vi "Upsampling for Reso Correction.vi"(9 "Insert Positions IN (for recursion)":i32[](array[numeric]), 10 "Extra points":i32, 11 "Pixel Map IN":i32[](array[numeric])) -> (2 "Insert Positions OUT":i32[](array[numeric]), 3 "Pixel Map OUT (Zoomed in)":i32[](array[numeric]))   [LabVIEW 2012]
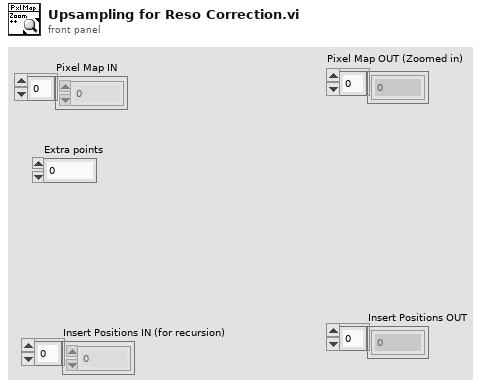
[diagram p1: front panel]
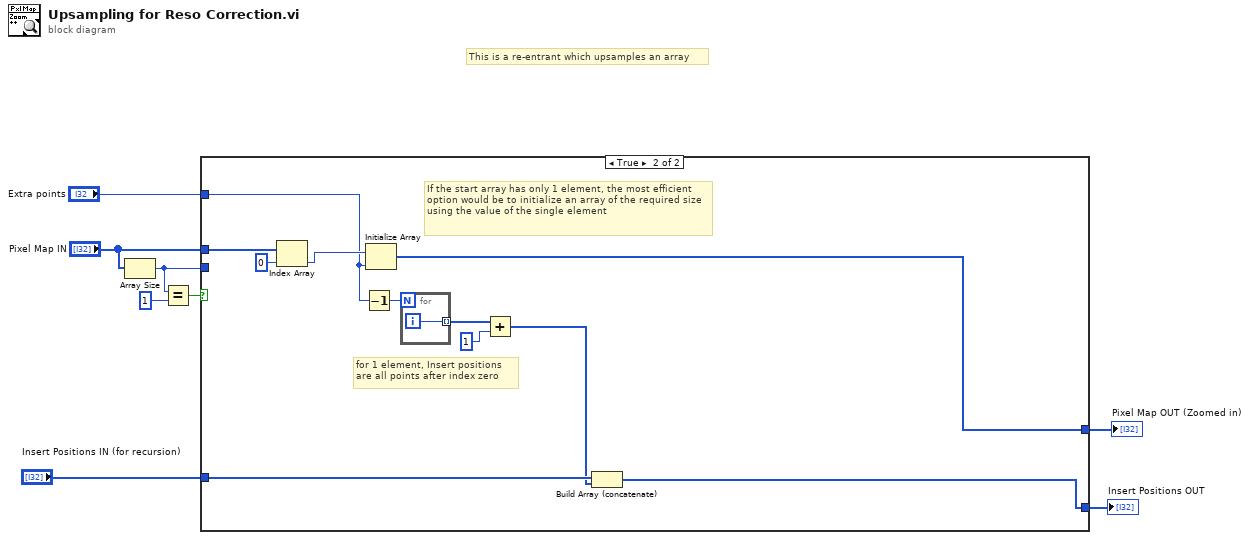
[diagram p0: block diagram]
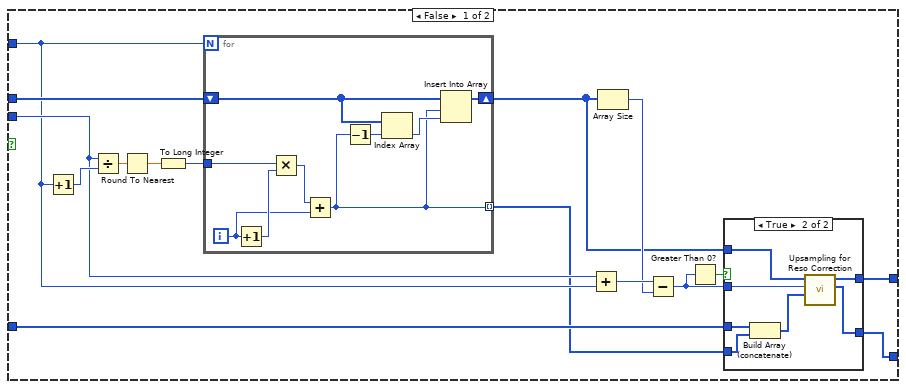
[diagram p2: hidden frame]
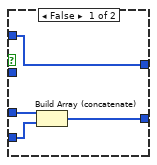
[diagram p3: hidden frame]
diagram:
  # "This is a re-entrant which upsamples an array"
  n1 = Array Size(array="Pixel Map IN") -> (size(s)=w5:i32)
  n2 = Equal?(x=w5, y=1) -> (x = y?=w3:bool)
  n3 = case shown="True" w3 {
    tunnel: w5 -> [w20 _]
    tunnel: "Pixel Map IN" -> [w14 w55]
    tunnel: "Extra points" -> [w13 w51]
    tunnel: [w12 w52] -> w6
    tunnel: [w9 w45] -> w2
    tunnel: "Insert Positions IN (for recursion)" -> [w11 w47]
    frame False {
      n4 = Increment(x=w13) -> (x+1=w24:i32)
      n5 = Divide(x=w20, y=w24) -> (x/y=w23:dbl)
      n6 = Round To Nearest(number=w23) -> (nearest integer value=w22:dbl)
      n7 = To Long Integer(number=w22) -> (32bit integer=w21:i32)
      n8 = for {
        N: w13 -> [_]
        shift-right: [w42] -> w15
        shift-left: w14 -> [w44]
        tunnel: w21 -> [w40]
        tunnel: [w36] -> w10 mode=indexing
        i -> [w38]
        n9 = Increment(x=w38) -> (x+1=w39:i32)
        n10 = Multiply(x=w40, y=w39) -> (x*y=w37:i32)
        n11 = Add(x=w37, y=w38) -> (x+y=w36:i32)
        n12 = Decrement(x=w36) -> (x-1=w41:i32)
        n13 = Index Array(array=w44, index=w41) -> (element=w43:i32)
        n14 = Insert Into Array(array=w44, index=w36, new element=w43) -> (w42:i32[])
      }
      n15 = Add(x=w20, y=w13) -> (x+y=w19:i32)
      n16 = Array Size(array=w15) -> (size(s)=w18:i32)
      n17 = Subtract(x=w19, y=w18) -> (x-y=w16:i32)
      n18 = Greater Than 0?(x=w16) -> (x > 0?=w17:bool)
      n19 = case shown="True" w17 {
        tunnel: w16 -> [_ w33]
        tunnel: w15 -> [w28 w35]
        tunnel: [w28 w34] -> w12
        tunnel: w11 -> [w27 w32]
        tunnel: w10 -> [w26 w31]
        tunnel: [w25 w29] -> w9
        frame False {
          n20 = Build Array (concatenate)(w27, w26) -> (w25:i32[])
        }
        frame True {
          n21 = Build Array (concatenate)(w32, w31) -> (w30:i32[])
          n22 = call "Upsampling for Reso Correction.vi"("Insert Positions IN (for recursion)"=w30, "Extra points"=w33, "Pixel Map IN"=w35) -> ("Insert Positions OUT"=w29:i32[], "Pixel Map OUT (Zoomed in)"=w34:i32[])  [unwired: 7 in]
        }
      }
    }
    frame True {
      # "for 1 element, Insert positions are all points after index zero"
      # "If the start array has only 1 element, the most efficient option would be to initialize an array of the required size using the value of the single element"
      n23 = Index Array(array=w55, index=0) -> (element=w53:i32)
      n24 = Decrement(x=w51) -> (x-1=w50:i32)
      n25 = Initialize Array(w53, w51) -> (w52:i32[])
      n26 = for {
        N: w50 -> [_]
        tunnel: [w56] -> w49 mode=indexing
        i -> [w56]
      }
      n27 = Add(x=w49, y=1) -> (x+y=w46:i32[])
      n28 = Build Array (concatenate)(w47, w46) -> (w45:i32[])
    }
  }
  "Pixel Map OUT (Zoomed in)" <- w6
  "Insert Positions OUT" <- w2
